vi "Write SV Data.vi"(8 "error in (no error)":errorcluster, 10 "SV Data":refnum<k21>="ni.var.psp://rt pxi target/PAS_Var/Data", 11 "PAS Control in":refnum<class "PAS Control.lvclass">) -> (0 "error out":errorcluster, 3 "PAS Control out":refnum<class "PAS Control.lvclass">)   [LabVIEW 2012, in "PAS Control.lvclass"]
uses:
  PAS Control.lvclass
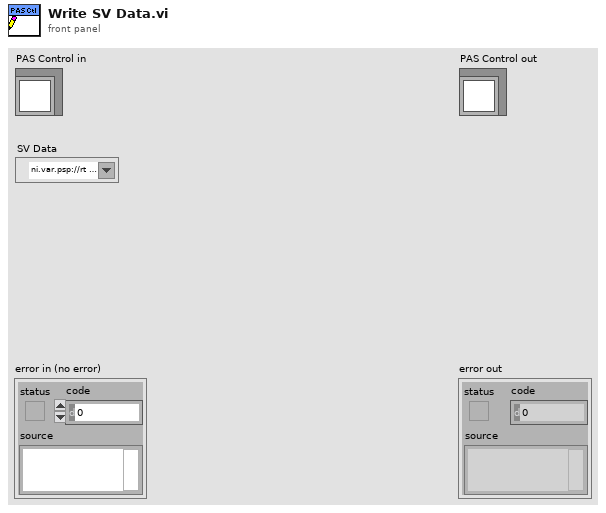
[diagram p1: front panel]
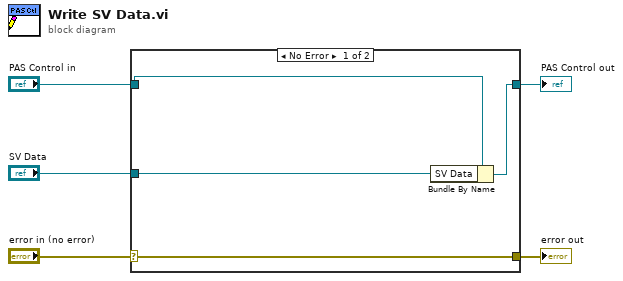
[diagram p0: block diagram]
diagram:
  n1 = case shown="No Error" "error in (no error)" {
    selector: "error in (no error)" -> [w9 w10]
    tunnel: [w9 w10] -> w4
    tunnel: [w7 w11] -> w2
    tunnel: "PAS Control in" -> [w8 w11]
    tunnel: "SV Data" -> [w6 _]
    frame No Error {
      n2 = Bundle By Name(cluster=w8, "SV Data"=w6) -> (w7:refnum<class "PAS Control.lvclass">)
    }
    frame Error {
    }
  }
  "error out" <- w4
  "PAS Control out" <- w2
